vi "TDF - Filter Signals (Classic).vi"(0 "reference in":refnum<class "GSwFormDSP.lvclass">, 5 "error in (no error)":errorcluster, 6 "Anotate Signal Name":bool=TRUE) -> (14 "reference in":refnum<class "GSwFormDSP.lvclass">, 19 "error out":errorcluster)   [LabVIEW 2020, in "GSwFormDSP.lvclass"]
uses:
  GSwFormDSP.lvclass
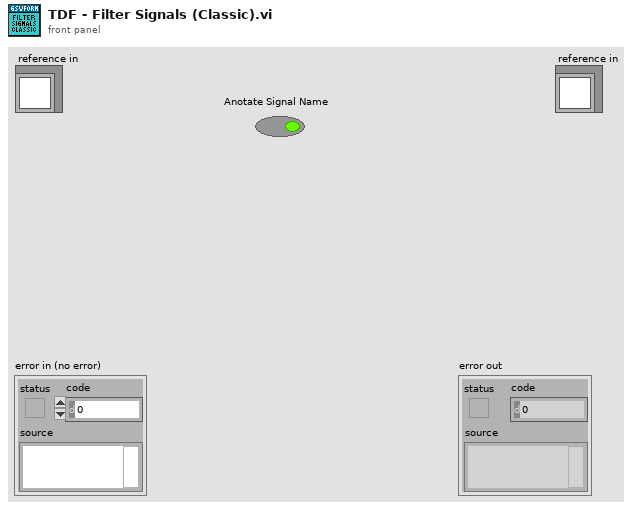
[diagram p1: front panel]
types:
  T1 = typedef "GSwFormDSP.lvclass/ObjectAttributes.ctl" = cluster{"Wform Ref":refnum<data-value>, "Nb Signals":i32, "Spectral Function Parameters":T2, "FFT":waveform(cdb)[], "Nb FFT":i32, "Nb Averages":i32[], "Reference Indexes":i32[], "Response Indexes":i32[], "Coherence":waveform(dbl)[], "TDF Parameters":T4, "DAQ":cluster{"Duration (sec)":dbl, "Buffer Size (Samples)":i32, "Offset (Samples)":i32}, "Filter Impulse Response (TDF)":waveform(dbl), "Sound Playback":T5}
  T2 = typedef "GSwFormDSP.lvclass/Spectral Parameters.ctl" = cluster{"Frequency resolution (Hz)":dbl, "Overlap":dbl, "Window":T3}
  T3 = typedef "NI_AALPro.lvlib/windowTd.ctl" = u32
  T4 = typedef "GSwFormDSP.lvclass/TDF Parameters.ctl" = cluster{"Filter":enum32{"Lowpass", "Highpass", "Bandpass", "Bandstop"}, "Type:":enum16{"Butterworth", "Chebyshev", "Inv Chebyshev", "Elliptic", "Bessel"}, "LP cutoff freq":dbl, "HP cutoff freq":dbl, "Order":i32, "passband ripple (dB)":dbl, "stopband attenuation (dB)":dbl, "Phaseless Filter":bool, "Include Fade IN and OUT":bool}
  T5 = typedef "GSwFormDSP.lvclass/Sound Playback.ctl" = cluster{"Timer start (ms)":u32, "task ID":T6, "Cursor Init Location (s)":dbl, "SC Volume":dbl}
  T6 = typedef "Sound Output Task ID.ctl" = u32
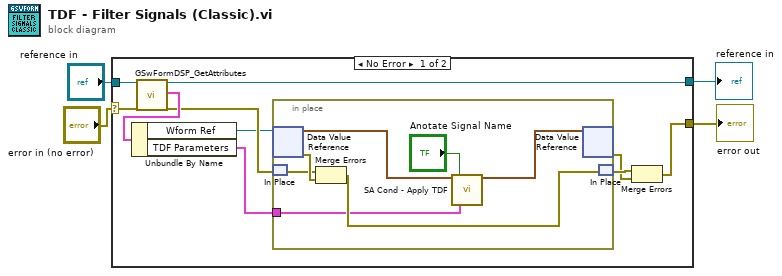
[diagram p0: block diagram]
diagram:
  n1 = case shown="No Error" "error in (no error)" {
    selector: "error in (no error)" -> [w12 w23]
    tunnel: [w14 w23] -> w3
    tunnel: [w10 w22] -> w2
    tunnel: "reference in" -> [w13 w22]
    frame No Error {
      n2 = call "GSwFormDSP_GetAttributes.vi"("reference in"=w13, "error in (no error)"=w12) -> ("reference out"=w10:refnum<class "GSwFormDSP.lvclass">, "attributes"=w11:T1, "error out"=w9:errorcluster)  [unwired: 14 in, 1 out]
      n3 = Unbundle By Name(w11) -> ("Wform Ref"=w8:refnum<data-value>, "TDF Parameters"=w7:T4)
      n4 = in-place {
        in-place-border: w7 -> [w15]
        n5 = in-place-dvr #1(w8) -> (w16:waveform(dbl)[], w19:errorcluster)
        n6 = in-place-match #2(w9) -> (w18:errorcluster)
        n7 = Merge Errors(w18, w19) -> (w20:errorcluster)
        n8 = call "SA Cond - Apply TDF.vi"("Signals IN"=w16, "Anotate Signal Name"="Anotate Signal Name", "TDF Parameters"=w15) -> ("Signals OUT"=w21:waveform(dbl)[])  [unwired: 16 in]
        n9 = in-place-dvr #1(w21) -> (w5:errorcluster)  [unwired: 1 out]
        n10 = in-place-match #2(w20) -> (w6:errorcluster)
      }
      n11 = Merge Errors(w6, w5) -> (w14:errorcluster)
    }
    frame Error {
    }
  }
  "error out" <- w3
  "reference in" <- w2
